vi "UVI_PopUp Menu_Create.vi"(0 "PopUpMenuItems":T2[](array[typedef]) {"uFlags" items=["MF_STRING"=0, "MF_GRAYED"=1, "MF_DISABLED"=2, "MF_CHECKED"=8, "MF_HILITE"=128, "MF_POPUP"=16, "MF_SEPARATOR"=2048]}, 5 "Menu params":T1, 7 "Mouse position":cluster{"x":i32, "y":i32}, 9 "Active Window handle":u32, 12 "Simple List":string[](array[string])) -> (6 "element":string, 15 "error out":errorcluster)   [LabVIEW 2013]
uses:
  TD_PopUp Menu_Items.ctl
  TD_PopUp Menu_Flags.ctl
  TD_PopUp Menu_Parameters.ctl
panel:
  in  "error in (no error)":errorcluster
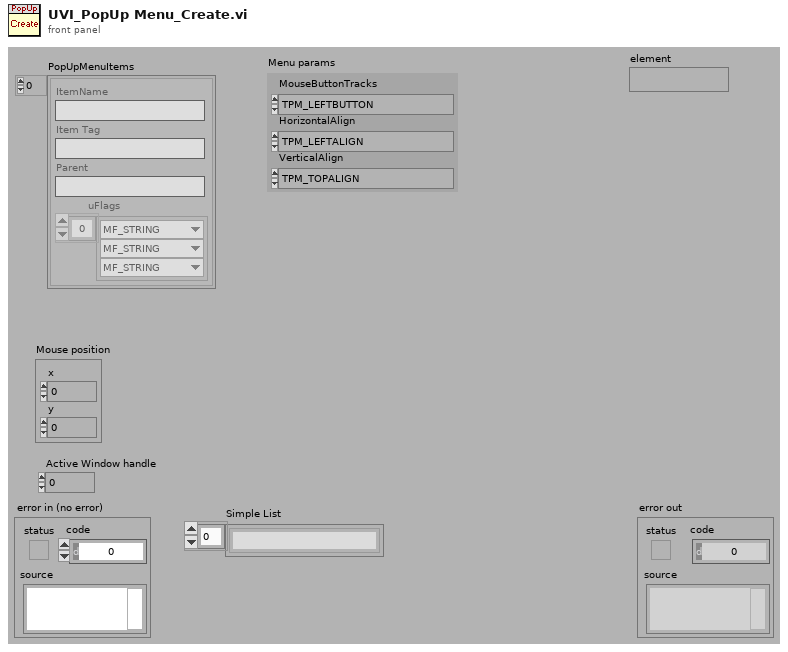
[diagram p1: front panel]
types:
  T1 = typedef "TD_PopUp Menu_Parameters.ctl" = cluster{"MouseButtonTracks":enum16{"TPM_LEFTBUTTON", "TPM_RIGHTBUTTON"}, "HorizontalAlign":enum16{"TPM_LEFTALIGN", "TPM_CENTRALALIGN", "TPM_RIGHTALIGN"}, "VerticalAlign":enum16{"TPM_TOPALIGN", "TPM_CENTRALALIGN", "TPM_BOTTOMALIGN"}}
  T2 = typedef "TD_PopUp Menu_Items.ctl" = cluster{"ItemName":string, "Item Tag":string, "Parent":string, "uFlags":T3[]}
  T3 = typedef "TD_PopUp Menu_Flags.ctl" = u32
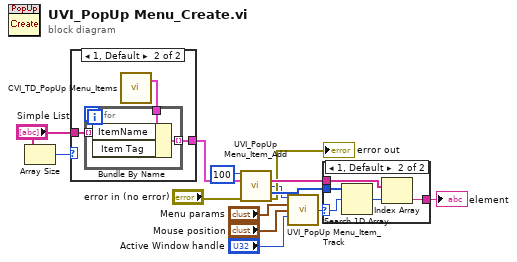
[diagram p0: block diagram]
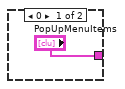
[diagram p2: hidden frame]
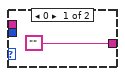
[diagram p3: hidden frame]
diagram:
  n1 = Array Size(array="Simple List") -> (size(s)=w3:i32)
  n2 = case shown="1, Default" w3 {
    tunnel: "Simple List" -> [_ w17]
    tunnel: ["PopUpMenuItems" w16] -> w1
    frame 0 {
    }
    frame 1, Default {
      n3 = call "CVI_TD_PopUp Menu_Items.vi"() -> (1:w18:T2)  [unwired: 1 out]
      n4 = for {
        tunnel: w18 -> [w21]
        tunnel: w17 -> [w20] mode=indexing
        tunnel: [w19] -> w16 mode=indexing
        n5 = Bundle By Name(cluster=w21, "ItemName"=w20, "Item Tag"=w20) -> (w19:T2)
      }
    }
  }
  n6 = call "UVI_PopUp Menu_Item_Add.vi"("StartIDItem"=100, "PopUpMenuItems"=w1, "error in (no error)"="error in (no error)") -> ("ItemTag"=w13:string[], "hMenu"=w4:u32, "ItemID"=w9:i32[], "error out"=→"error out":errorcluster)  [unwired: 1 in, 8 out]
  n7 = call "UVI_PopUp Menu_Item_Track.vi"("hMenu"=w4, "Menu params"="Menu params", "Mouse position"="Mouse position", "Active Window handle"="Active Window handle") -> ("MenuSelection"=w12:u32)  [unwired: 1 in, 10 out]
  n8 = case shown="1, Default" w12 {
    selector: w12 -> [_ w24]
    tunnel: w13 -> [_ w27]
    tunnel: ["" w26] -> w11
    tunnel: w9 -> [_ w25]
    frame 0 {
    }
    frame 1, Default {
      n9 = Search 1D Array(1D array=w25, element=w24) -> (index of element=w23:i32)  [unwired: 1 out]
      n10 = Index Array(array=w27, index=w23) -> (element=w26:string)
    }
  }
  "element" <- w11
